vi "WRP Validate.vi"(7 "kineticEnergy":dbl, 8 "error in (no error)":errorcluster, 9 "passEnergy":dbl, 10 "lensMode":string, 11 "elementSet":string) -> (0 "error out":errorcluster, 3 "function return":i32)   [LabVIEW 2018, in "SesWrapper.lvlib"]
doc: "int STDCALL WRP_Validate(const String elementSet, const String lensMode, double passEnergy, double kineticEnergy);"
uses:
  SesWrapper.lvlib
  build/Debug/SESWrapper.dll
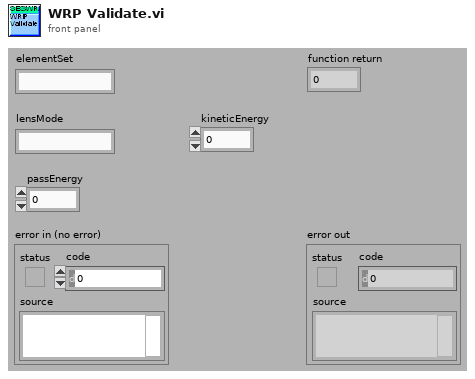
[diagram p1: front panel]
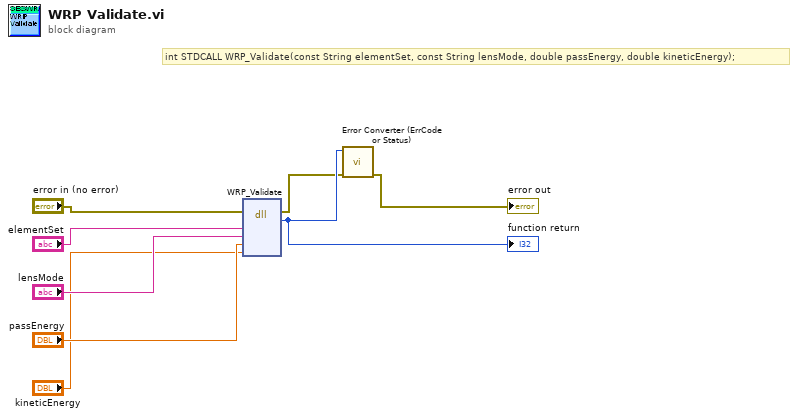
[diagram p0: block diagram]
diagram:
  # "int STDCALL WRP_Validate(const String elementSet, const String lensMode, double passEnergy, double kineticEnergy);"
  n1 = dll-call lib="C:/Development/svn/seswrapper-lib/build/Debug/SESWrapper.*" fn="WRP_Validate"(error in="error in (no error)", "elementSet"="elementSet", "lensMode"="lensMode", "passEnergy"="passEnergy", "kineticEnergy"="kineticEnergy") -> (error out=w2:errorcluster, w8:i32)  [unwired: 6 in, 1 out]
  "function return" <- w8
  n2 = call "Error Converter (ErrCode or Status).vi"("error in (no error)"=w2, "error code"=w8) -> ("error out"=→"error out":errorcluster)  [unwired: 9 in]
